vi "Insert Replacement String.vi"(6 "length to replace":i32, 9 "offset of replacement (0)":i32, 10 "substring":string, 11 "string":string) -> (3 "result string":string)   [LabVIEW 2020]
panel:
  out "replaced substring":string
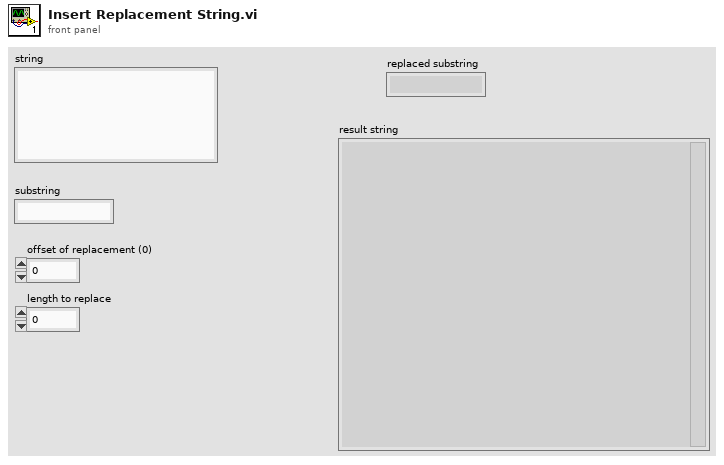
[diagram p1: front panel]
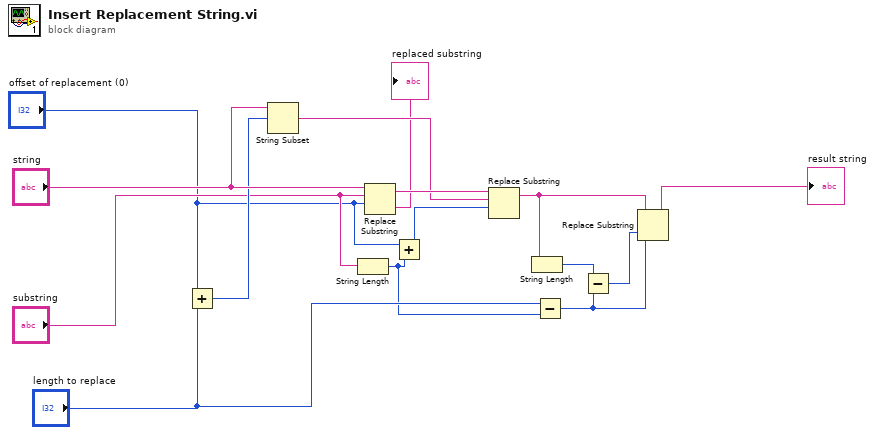
[diagram p0: block diagram]
diagram:
  n1 = Add(x="offset of replacement (0)", y="length to replace") -> (x+y=w14:i32)
  n2 = String Subset(string="string", offset (0)=w14) -> (substring=w12:string)  [unwired: 1 in]
  n3 = String Length(string="substring") -> (length=w7:i32)
  n4 = Replace Substring(3:"offset of replacement (0)", 4:"substring", 5:"string") -> (0:→"replaced substring":string, 1:w13:string)  [unwired: 1 in]
  n5 = Add(x="offset of replacement (0)", y=w7) -> (x+y=w9:i32)
  n6 = Replace Substring(3:w9, 4:w12, 5:w13) -> (1:w6:string)  [unwired: 1 in, 1 out]
  n7 = String Length(string=w6) -> (length=w5:i32)
  n8 = Subtract(x="length to replace", y=w7) -> (x-y=w3:i32)
  n9 = Subtract(x=w5, y=w3) -> (x-y=w4:i32)
  n10 = Replace Substring(2:w3, 3:w4, 5:w6) -> (1:→"result string":string)  [unwired: 1 in, 1 out]
